vi "Autonomous Independent.vi"() -> ()   [LabVIEW 2018]
doc: "This VI is called when autonomous begins, and will automatically be terminated when autonomous ends. You can carry out timed or sensor driven robot movement independently without needing to return to the caller."
uses:
  TypeDefs/typedef_enum_Refnums.ctl
  TypeDefs/Joystick Buttons.ctl
  <vilib>/Rock Robotics/WPI/Utilities/WPI_GetSetVariantRefNum.vi
  <vilib>/Rock Robotics/Network Tables/NT Read String.vi
  <vilib>/Rock Robotics/Network Tables/NT Write Numeric Array.vi
  <vilib>/Rock Robotics/WPI/DriverStation/WPI_DriverStationDerivedRobotMode.ctl
  <vilib>/ptbypt/NI_PtbyPt.lvlib
panel:
  in  "default do nothingsdf":cluster{"Waypoints":dbl[][], "Reverse?":bool}[](array[cluster])=[{"Waypoints"=[[0.0, 0.0], [-2.0, 25000.0], [-19964.0, 25172.0]], "Reverse?"=TRUE}, {"Waypoints"=[[0.0, 0.0], [-2.0, 10416.0], [-13020.0, 31248.0], [-35248.0, 58740.0]], "Reverse?"=FALSE}]
  in  "Left Level 1 to Left Rocket":cluster{"Waypoints":dbl[][], "Reverse?":bool}[](array[cluster])=[{"Waypoints"=[[0.0, 0.0], [-2.0, 20832.0], [-18436.0, 41664.0], [-35000.0, 70000.0]], "Reverse?"=FALSE}]
  in  "Left Level 1 to Left Cargo":cluster{"Waypoints":dbl[][], "Reverse?":bool}[](array[cluster])=[{"Waypoints"=[[0.0, 0.0], [2.0, 20832.0], [19240.0, 36248.0], [19280.0, 65000.0]], "Reverse?"=FALSE}]
  in  "Second Path that we currently don't use":cluster{"Waypoints":dbl[][], "Reverse?":bool}[](array[cluster])=[{"Waypoints"=[[0.0, 0.0], [-2.0, 25000.0], [-19964.0, 25172.0]], "Reverse?"=TRUE}, {"Waypoints"=[[0.0, 0.0], [-2.0, 10416.0], [-13020.0, 31248.0], [-35248.0, 58740.0]], "Reverse?"=FALSE}]
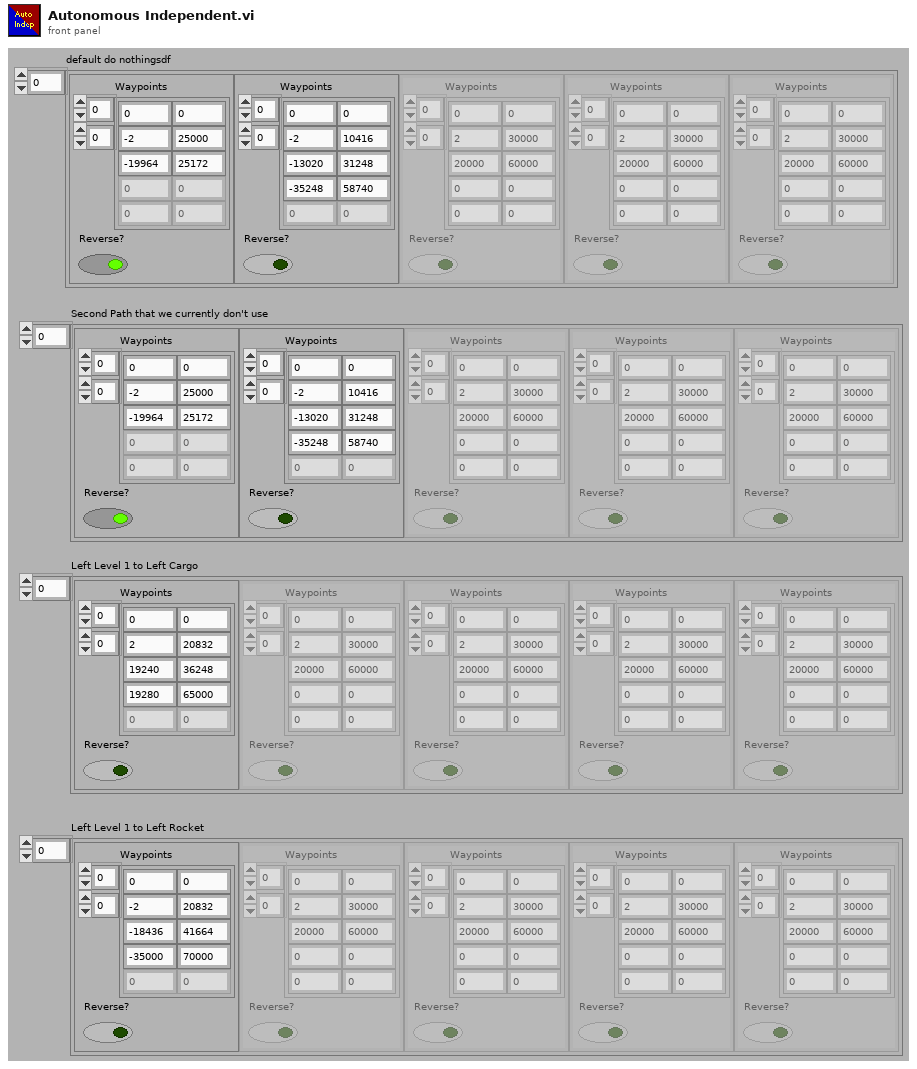
[diagram p1: front panel]
types:
  T1 = typedef "WPI_JoystickDevRef.ctl" = cluster{"Device":T2}
  T2 = typedef "WPI_JoystickDeviceEnum.ctl" = enum16{"USB 0", "USB 1", "USB 2", "USB 3", "USB 4", "USB 5"}
  T3 = typedef "WPI_DriverStationDerivedRobotMode.ctl" = enum16{"Init", "Execute", "Stop"}
  T4 = typedef "Joystick Buttons.ctl" = enum16{"Trigger", "Thumb", "Top 3", "Top 4", "Top 5", "Top 6", "Bottom 7", "Bottom 8", "Bottom 9", "Bottom 10", "Bottom 11", "Bottom 12"}
  T5 = typedef "typedef_enum_Refnums.ctl" = enum16{"Ball_Encoder", "Ball_Motor", "Camera", "Linefollow_3", "Linefollow_2", "Linefollow_1", "Gyro", "Hatch_Solenoid", "Climb_Back_Solenoid", "Arm_Encoder", "Arm_Motor", "Lift_Encoder", "Drive", "Drive_Motor_R", "Drive_Motor_L", "Drive_Encoder_R", "Drive_Encoder_L", "Joy_R", "Joy_L", "Wrist_Motor", "Wrist_Encoder", "Climb Upper Limit", "Climb Lower Limit ", "Climb_Front_Motor"}
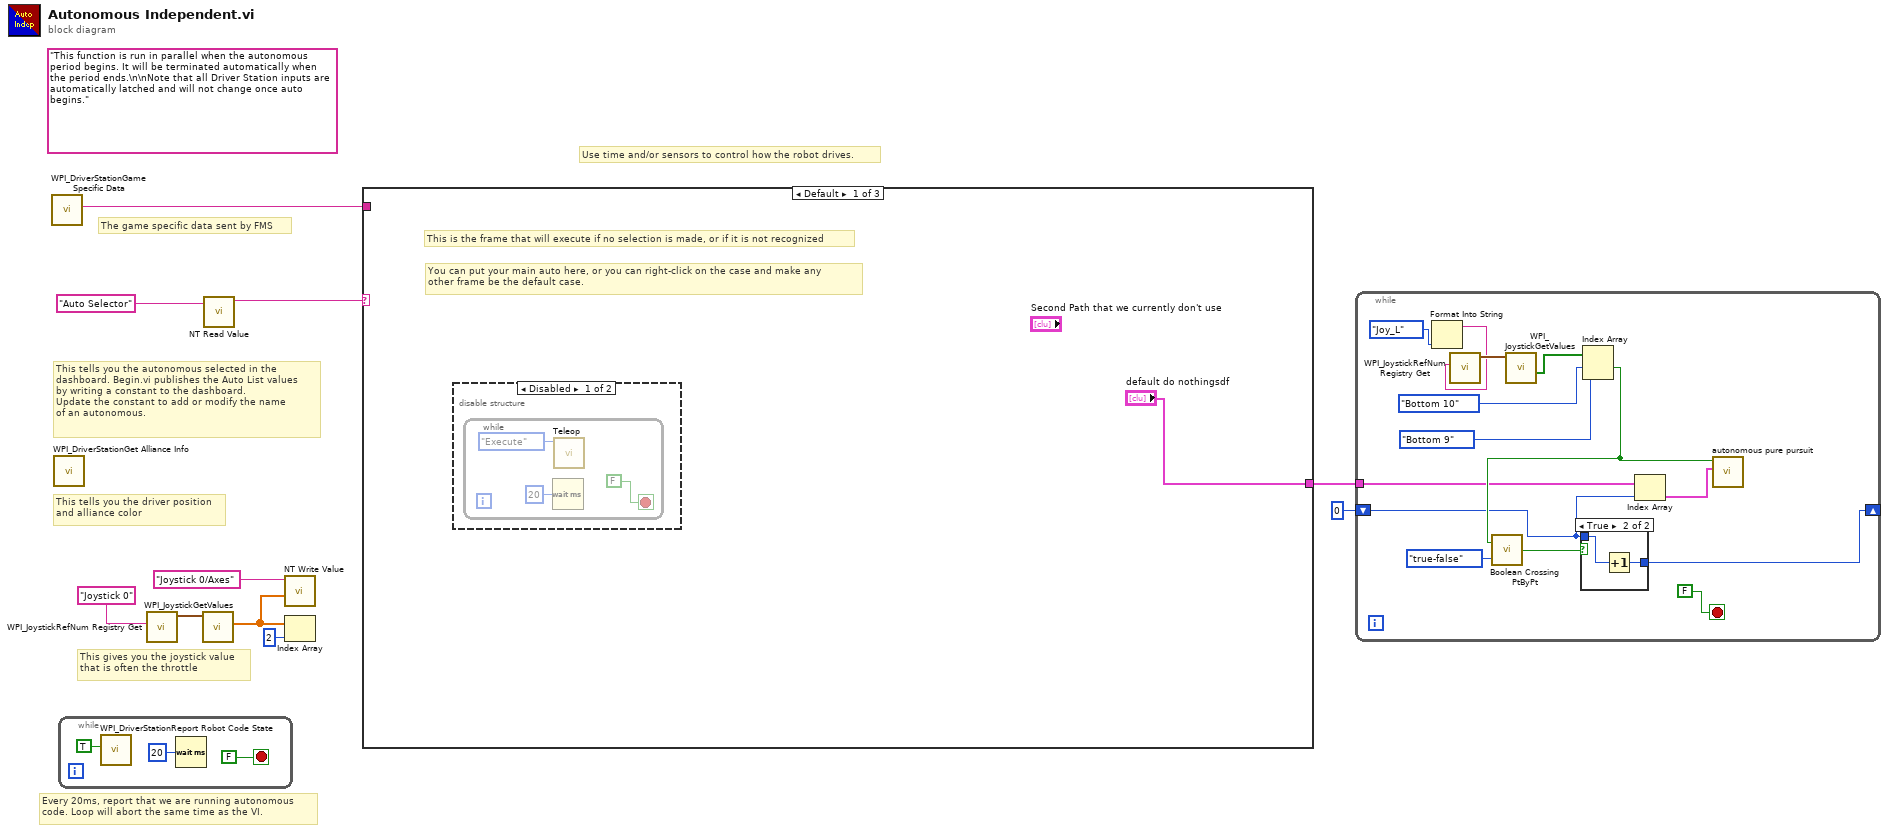
[diagram p0: block diagram]
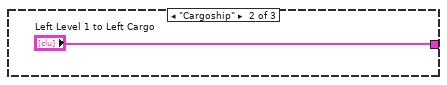
[diagram p4: hidden frame]
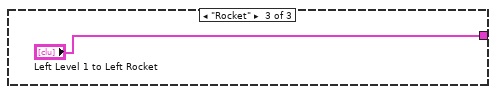
[diagram p5: hidden frame]
diagram:
  (unwired) "This function is run in parallel when the autonomous period begins. It will be terminated automatically when the period ends.\n\nNote that all Driver Station inputs are automatically latched and will not change once auto begins."
  # "The game specific data sent by FMS"
  # "This tells you the autonomous selected in the \ndashboard. Begin.vi publishes the Auto List values\nby writing a constant to the dashboard.\nUpdate the constant to add or modify the name\nof an autonomous."
  # "Every 20ms, report that we are running autonomous\ncode. Loop will abort the same time as the VI."
  # "This gives you the joystick value\nthat is often the throttle"
  # "Use time and/or sensors to control how the robot drives."
  # "This tells you the driver position\nand alliance color"
  n1 = call <vilib>:"WPI_DriverStationGame Specific Data.vi"() -> ("Game Specific Data"=w3:string)  [unwired: 11 in]
  n2 = call <vilib>:"WPI_DriverStationGet Alliance Info.vi"() -> ()  [unwired: 12 out]
  n3 = while {
    stop <- FALSE stop-if-true
    n4 = call <vilib>:"WPI_DriverStationReport Robot Code State.vi"("Autonomous"=TRUE) -> ()  [unwired: 10 in, 1 out]
    n5 = Wait (ms)(milliseconds to wait=u32 20) -> ()  [unwired: 1 out]
  }
  n6 = call <vilib>:"WPI_JoystickRefNum Registry Get.vi"("refnum name"="Joystick 0") -> ("JoystickDevRef"=w9:T1)  [unwired: 1 in, 9 out]
  n7 = call <vilib>:"WPI_JoystickGetValues.vi"("JoystickDevRef"=w9) -> ("Axes"=w5:dbl[])  [unwired: 6 in, 4 out]
  n8 = call-poly <vilib>:"NT Read Value.vi"("Name"="Auto Selector") -> ("String"=w6:string)  [unwired: 9 in, 1 out]
  n9 = call-poly <vilib>:"NT Write Value.vi"("Numeric Array"=w5, "Name"="Joystick 0/Axes") -> ()  [unwired: 9 in, 1 out]
  n10 = Index Array(array=w5, index=2) -> ()  [unwired: 1 out]
  n11 = case shown="Default" w6 {
    tunnel: w3 -> [_ _ _]
    tunnel: ["default do nothingsdf" "Left Level 1 to Left Cargo" "Left Level 1 to Left Rocket"] -> w1
    frame Default {
      # "You can put your main auto here, or you can right-click on the case and make any\nother frame be the default case."
      # "This is the frame that will execute if no selection is made, or if it is not recognized"
      n12 = disable-structure shown="Disabled" {
        frame Disabled {
          n13 = while {
            stop <- FALSE stop-if-true
            n14 = Wait (ms)(milliseconds to wait=u32 20) -> ()  [unwired: 1 out]
            n15 = call "Teleop.vi"("Call Context"=WPI_DriverStationDerivedRobotMode."Execute") -> ()  [unwired: 11 in]
          }
        }
        frame Enabled {
        }
      }
    }
    frame "Cargoship" {
    }
    frame "Rocket" {
    }
  }
  n16 = while {
    shift-right: [w23] -> _
    shift-left: 0 -> [w22]
    tunnel: w1 -> [w20]
    stop <- FALSE stop-if-true
    n17 = Format Into String(typedef_enum_Refnums."Joy_L" ("RefNums")) -> (resulting string=w30:string)  [unwired: 3 in, 1 out]
    n18 = call <vilib>:"WPI_JoystickRefNum Registry Get.vi"("refnum name"=w30) -> ("JoystickDevRef"=w32:T1)  [unwired: 1 in, 9 out]
    n19 = call <vilib>:"WPI_JoystickGetValues.vi"("JoystickDevRef"=w32) -> ("Buttons"=w28:bool[])  [unwired: 6 in, 4 out]
    n20 = Index Array(array=w28, index #1=Joystick_Buttons."Bottom 10" ("Enum"), index #2=Joystick_Buttons."Bottom 9" ("Enum")) -> (element #1=w26:bool)  [unwired: 1 out]
    n21 = call <vilib>:"Boolean Crossing PtByPt.vi"("direction"=enum16{"either", "false-true", "true-false"}."true-false", "input"=w26) -> ("crossing"=w24:bool)  [unwired: 1 in]
    n22 = case shown="True" w24 {
      tunnel: w22 -> [w34 w36]
      tunnel: [w34 w35] -> w23
      frame False {
      }
      frame True {
        n23 = Increment(x=w36) -> (x+1=w35:i32)
      }
    }
    n24 = Index Array(array=w20, index=w22) -> (element=w21:cluster{"Waypoints":dbl[][], "Reverse?":bool})
    n25 = call "autonomous pure pursuit.vi"("Waypoint Data"=w21, "Button"=w26) -> ()  [unwired: 10 in]
  }
